vi "MGI Non-Uniform B-Spline.vi"(6 "Weights[]":dbl[](array[numeric])=[0.25, 0.25, 0.25, 0.25, 0.25, 0.25, 0.25, 0.25, 0.25], 7 "Degree":i32=5, 8 "u":dbl=41.7451, 9 "Knot Multiplicities[]":i32[](array[numeric])=[6, 3, 6], 10 "Knots[]":dbl[](array[numeric])=[0.0, 5.69376337762, 41.7451953785], 11 "Control Points[][]":dbl[][](array[numeric])=[[381.5453186035156, -17.001089096069336, 123.35271453857422], [381.5005798339844, -17.00055503845215, 123.34944152832031], [381.4560241699219, -17.000045776367188, 123.34617614746094], [381.1888427734375, -16.99648094177246, 123.32664489746094], [380.8610534667969, -16.992168426513672, 123.30262756347656], [380.5331115722656, -16.987791061401367, 123.27851104736328], [380.2501525878906, -16.984203338623047, 123.2575912475586], [379.96710205078125, -16.980527877807617, 123.23660278320312], [379.68402099609375, -16.976825714111328, 123.21554565429688]]) -> (3 "C(u)":dbl[](array[numeric]))   [LabVIEW 2020]
doc: "Calculate a Non-uniform rational B-Spline curve value. Input is formatted for compatibility with a STEP file (ISO-10303).\n\nAuthored by Thomas E. Henage\nsupport@mooregoodideas.com\nwww.mooregoodideas.com\n\nCopyright (c) 2010, Moore Good Ideas, Inc.\n\nAll rights reserved.\n\nRedistribution and use in source and binary forms, with or without modification, are permitted provided that the following conditions are met:\n\n * Redistributions of source code must retain the above copyright notice, this list of conditions and the following disclaimer.\n * Redistributions in binary form must reproduce the above copyright notice, this list of conditions and the following disclaimer in the documentation and/or other materials provided with the distribution.\n * Neither the name of Moore Good Ideas, Inc. nor the names of its contributors may be used to endorse or promote products derived from this software without specific prior written permission.\n\nTHIS SOFTWARE IS PROVIDED BY THE COPYRIGHT HOLDERS AND CONTRIBUTORS \"AS IS\" AND ANY EXPRESS OR IMPLIED WARRANTIES, INCLUDING, BUT NOT LIMITED TO, THE IMPLIED WARRANTIES OF MERCHANTABILITY AND FITNESS FOR A PARTICULAR PURPOSE ARE DISCLAIMED. IN NO EVENT SHALL THE COPYRIGHT OWNER OR CONTRIBUTORS BE LIABLE FOR ANY DIRECT, INDIRECT, INCIDENTAL, SPECIAL, EXEMPLARY, OR CONSEQUENTIAL DAMAGES (INCLUDING, BUT NOT LIMITED TO, PROCUREMENT OF SUBSTITUTE GOODS OR SERVICES; LOSS OF USE, DATA, OR PROFITS; OR BUSINESS INTERRUPTION) HOWEVER CAUSED AND ON ANY THEORY OF LIABILITY, WHETHER IN CONTRACT, STRICT LIABILITY, OR TORT (INCLUDING NEGLIGENCE OR OTHERWISE) ARISING IN ANY WAY OUT OF THE USE OF THIS SOFTWARE, EVEN IF ADVISED OF THE POSSIBILITY OF SUCH DAMAGE."
panel:
  out "N(i,n,u)":dbl[][](array[numeric])
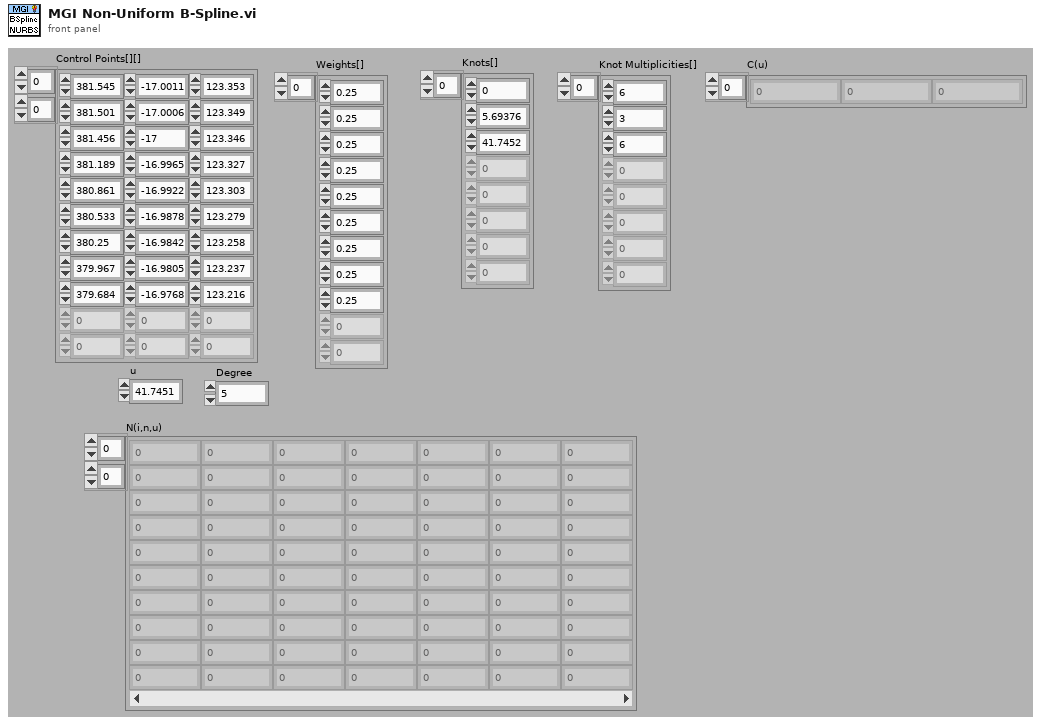
[diagram p1: front panel]
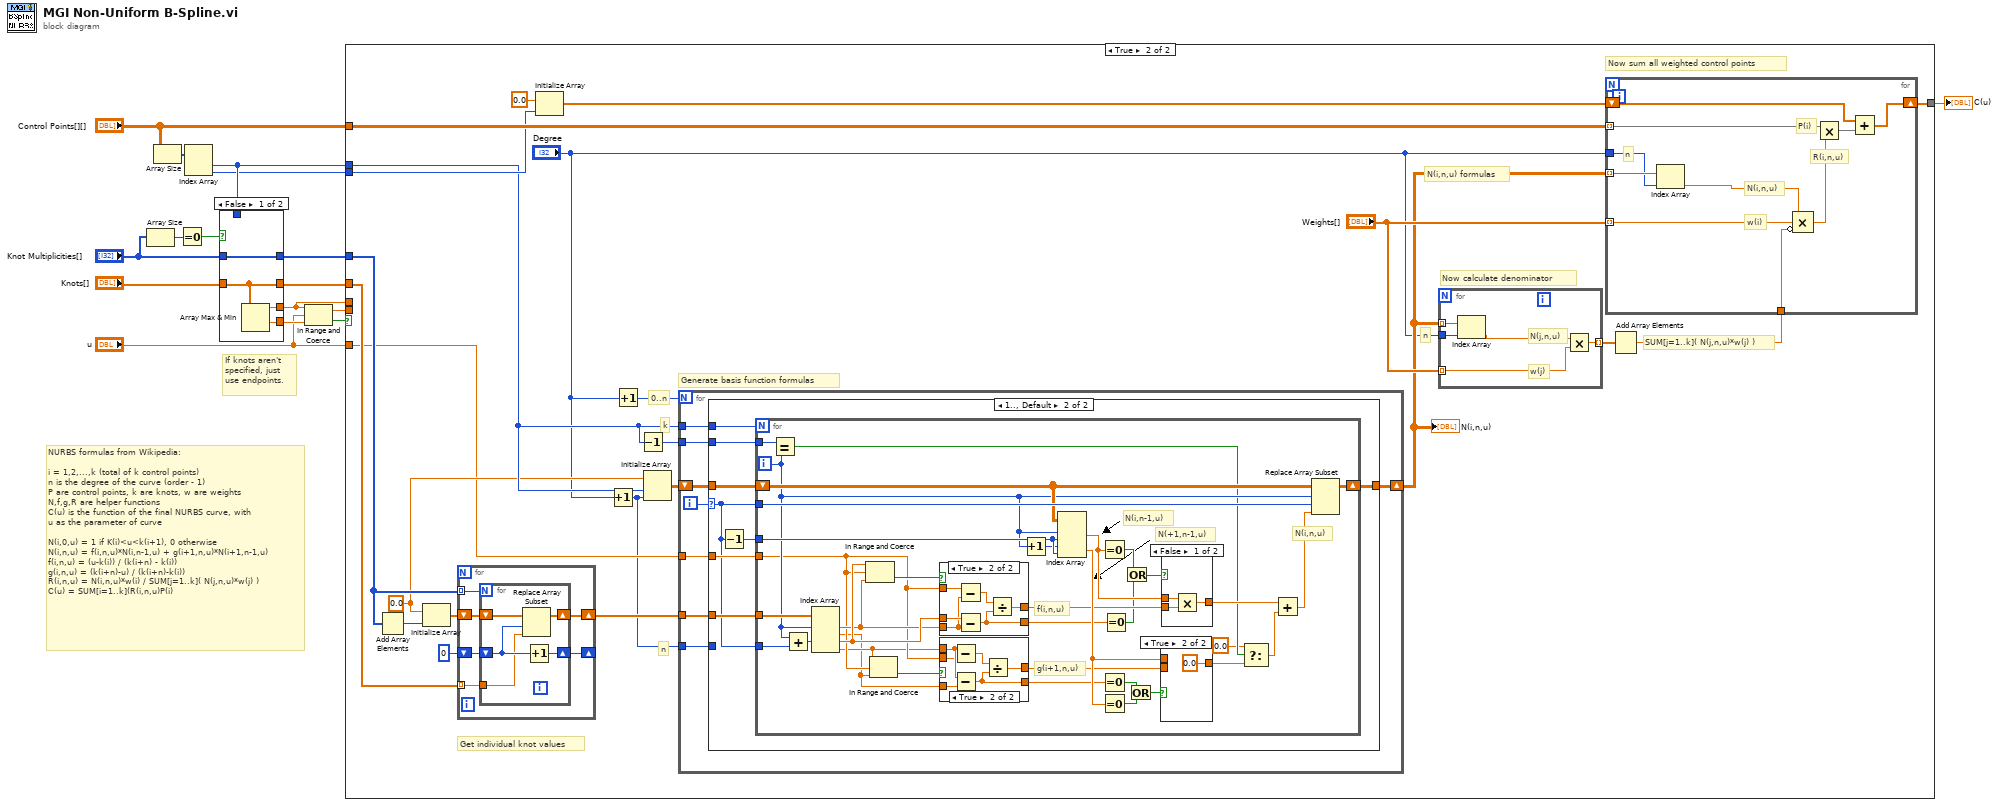
[diagram p0: block diagram]
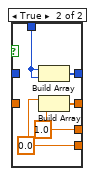
[diagram p2: hidden frame]
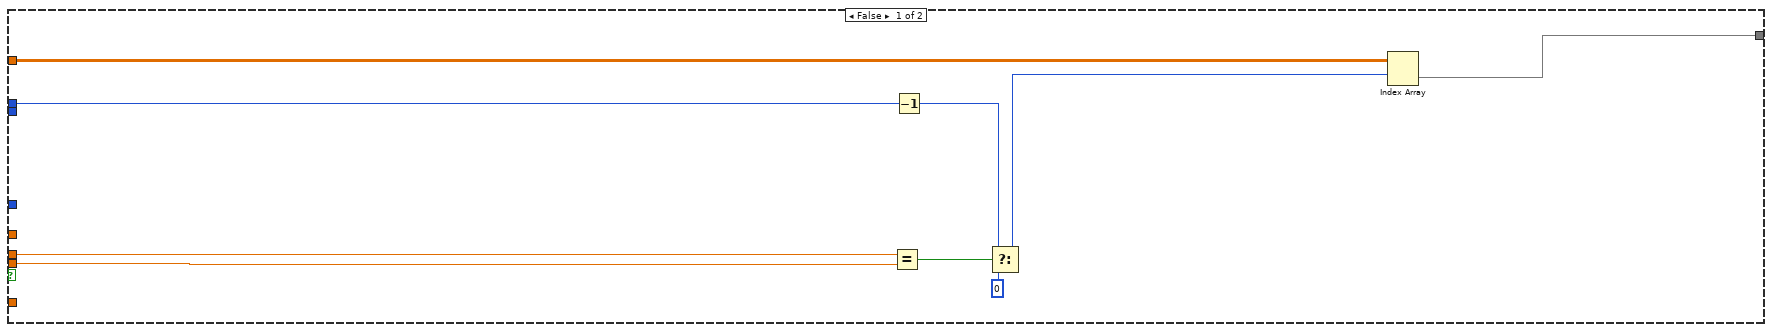
[diagram p3: hidden frame]
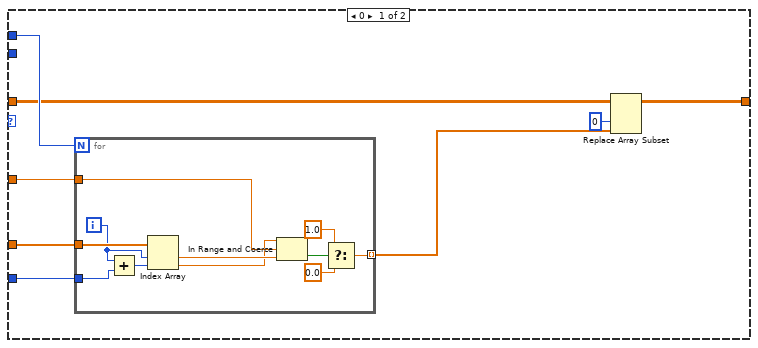
[diagram p4: hidden frame]
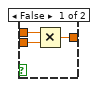
[diagram p7: hidden frame]
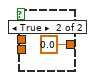
[diagram p8: hidden frame]
diagram:
  # "NURBS formulas from Wikipedia:\n\ni = 1,2,...,k (total of k control points)\nn is the degree of the curve (order - 1)\nP are control points, k are knots, w are weights\nN,f,g,R are helper functions\nC(u) is the function of the final NURBS curve, with\nu as the parameter of curve\n\nN(i,0,u) = 1 if K(i)<u<k(i+1), 0 otherwise\nN(i,n,u) = f(i,n,u)*N(i,n-1,u) + g(i+1,n,u)*N(i+1,n-1,u)\nf(i,n,u) = (u-k(i)) / (k(i+n) - k(i))\ng(i,n,u) = (k(i+n)-u) / (k(i+n)-k(i))\nR(i,n,u) = N(i,n,u)*w(i) / SUM[j=1..k]( N(j,n,u)*w(j) )\nC(u) = SUM[i=1..k](R(i,n,u)P(i)"
  # "If knots aren't\nspecified, just\nuse endpoints."
  n1 = Array Size(array="Knot Multiplicities[]") -> (size(s)=w4:i32)
  n2 = Array Size(array="Control Points[][]") -> (size(s)=w10:i32[])
  n3 = Equal To 0?(x=w4) -> (x = 0?=w3:bool)
  n4 = Index Array(array=w10) -> (element #1=w6:i32, element #2=w2:i32)  [unwired: 2 in]
  n5 = case shown="False" w3 {
    tunnel: "Knots[]" -> [w17 _]
    tunnel: [w20 w24] -> w16
    tunnel: [w19 w25] -> w12
    tunnel: "Knot Multiplicities[]" -> [w18 _]
    tunnel: [w18 w21] -> w8
    tunnel: [w17 w23] -> w7
    tunnel: w6 -> [_ w22]
    frame False {
      n6 = Array Max & Min(array=w17) -> (max value=w19:dbl, min value=w20:dbl)  [unwired: 2 out]
    }
    frame True {
      w24 = 0.0
      w25 = 1.0
      n7 = Build Array(w22, w22) -> (w21:i32[])
      n8 = Build Array(w24, w25) -> (w23:dbl[])
    }
  }
  n9 = In Range and Coerce(upper limit=w12, x="u", lower limit=w16) -> (coerced(x)=w13:dbl, In Range?=w14:bool)
  n10 = case shown="True" w14 {
    tunnel: w7 -> [_ w48]
    tunnel: "u" -> [_ w37]
    tunnel: w13 -> [w34 _]
    tunnel: w12 -> [w33 _]
    tunnel: "Control Points[][]" -> [w32 w57]
    tunnel: [w31 w53] -> w11
    tunnel: w6 -> [w30 w47]
    tunnel: w8 -> [_ w44]
    tunnel: w2 -> [_ w56]
    frame False {
      n11 = Equal?(x=w33, y=w34) -> (x = y?=w29:bool)
      n12 = Decrement(x=w30) -> (x-1=w28:i32)
      n13 = Select(t=w28, s=w29, f=0) -> (s? t:f=w26:i32)
      n14 = Index Array(array=w32, index (row)=w26) -> (element=w31:dbl[])  [unwired: 1 in]
    }
    frame True {
      w38 = 0.0
      # "Get individual knot values"
      # "n"
      # "0..n"
      # "k"
      # "Now sum all weighted control points"
      # "Now calculate denominator"
      # "Generate basis function formulas"
      # "n"
      # "SUM[j=1..k]( N(j,n,u)*w(j) )"
      # "N(i,n,u) formulas"
      n15 = Add Array Elements(numeric array=w44) -> (sum=w42:i32)
      n16 = Initialize Array(w38, w42) -> (w43:dbl[])
      n17 = for {
        tunnel: w48 -> [w63] mode=indexing
        tunnel: w44 -> [w62] mode=indexing
        shift-right: [w60] -> w40
        shift-left: w43 -> [w61]
        shift-right: [w58] -> _
        shift-left: 0 -> [w59]
        n18 = for {
          N: w62 -> [_]
          tunnel: w63 -> [w64]
          shift-right: [w67] -> w60
          shift-left: w61 -> [w68]
          shift-right: [w65] -> w58
          shift-left: w59 -> [w66]
          n19 = Replace Array Subset(array=w68, new element=w64, index=w66) -> (w67:dbl[])
          n20 = Increment(x=w66) -> (x+1=w65:i32)
        }
      }
      n21 = Initialize Array(0.0 ("element"), w56) -> (w54:dbl[])
      n22 = Increment(x="Degree") -> (x+1=w35:i32)
      n23 = Increment(x="Degree") -> (x+1=w45:i32)
      n24 = Decrement(x=w47) -> (x-1=w46:i32)
      n25 = Initialize Array(w38, w47, w35) -> (w49:dbl[][])
      n26 = for {
        N: w45 -> [_]
        shift-right: [w72] -> w39
        shift-left: w49 -> [w75]
        tunnel: w40 -> [w74]
        tunnel: w47 -> [w73]
        tunnel: w46 -> [w71]
        tunnel: w37 -> [w70]
        tunnel: w35 -> [w69]
        i -> [w76]
        n27 = case shown="1.., Default" w76 {
          selector: w76 -> [_ w96]
          tunnel: w75 -> [w81 w103]
          tunnel: w74 -> [w83 w99]
          tunnel: w73 -> [w84 w102]
          tunnel: [w80 w101] -> w72
          tunnel: w71 -> [_ w100]
          tunnel: w70 -> [w82 w97]
          tunnel: w69 -> [w77 _]
          frame 0 {
            n28 = for {
              N: w84 -> [_]
              tunnel: w83 -> [w95]
              tunnel: w77 -> [w94]
              tunnel: w82 -> [w93]
              tunnel: [w87] -> w79 mode=indexing
              i -> [w85]
              n29 = Add(x=w85, y=w94) -> (x+y=w86:i32)
              n30 = Index Array(array=w95, index #1=w85, index #2=w86) -> (element #1=w92:dbl, element #2=w91:dbl)
              n31 = In Range and Coerce(upper limit=w91, x=w93, lower limit=w92) -> (In Range?=w90:bool)  [unwired: 1 out]
              n32 = Select(t=1.0, s=w90, f=0.0) -> (s? t:f=w87:dbl)
            }
            n33 = Replace Array Subset(array=w81, new element=w79, index (col)=0 ("disabled index (col)")) -> (w80:dbl[][])  [unwired: 1 in]
          }
          frame 1.., Default {
            n34 = Decrement(x=w96) -> (x-1=w98:i32)
            n35 = for {
              N: w102 -> [_]
              shift-right: [w135] -> w101
              shift-left: w103 -> [w133]
              tunnel: w100 -> [w138]
              tunnel: w99 -> [w137]
              tunnel: w96 -> [w134]
              tunnel: w98 -> [w132]
              tunnel: w96 -> [w129]
              tunnel: w97 -> [w107]
              i -> [w131]
              # "g(i+1,n,u)"
              # "f(i,n,u)"
              # "N(+1,n-1,u)"
              # "N(i,n,u)"
              # "N(i,n-1,u)"
              n36 = Equal?(x=w138, y=w131) -> (x = y?=w125:bool)
              n37 = Add(x=w131, y=w129) -> (x+y=w136:i32)
              n38 = Index Array(array=w137, index #1=w131, index #3=w136) -> (element #1=w109:dbl, element #2=w105:dbl, element #3=w110:dbl, element #4=w106:dbl)  [unwired: 2 in]
              n39 = In Range and Coerce(upper limit=w110, x=w107, lower limit=w109) -> (In Range?=w108:bool)  [unwired: 1 out]
              n40 = In Range and Coerce(upper limit=w106, x=w107, lower limit=w105) -> (In Range?=w104:bool)  [unwired: 1 out]
              n41 = case shown="True" w108 {
                tunnel: [_ w149] -> w118
                tunnel: [_ w148] -> w112
                tunnel: w107 -> [_ w147]
                tunnel: w110 -> [_ w146]
                tunnel: w109 -> [_ w145]
                frame False {
                }
                frame True {
                  n42 = Subtract(x=w147, y=w145) -> (x-y=w150:dbl)
                  n43 = Subtract(x=w146, y=w145) -> (x-y=w148:dbl)
                  n44 = Divide(x=w150, y=w148) -> (x/y=w149:dbl)
                }
              }
              n45 = case shown="True" w104 {
                tunnel: w106 -> [_ w144]
                tunnel: w105 -> [_ w143]
                tunnel: [_ w141] -> w115
                tunnel: [_ w140] -> w111
                tunnel: w107 -> [_ w139]
                frame False {
                }
                frame True {
                  n46 = Subtract(x=w144, y=w139) -> (x-y=w142:dbl)
                  n47 = Subtract(x=w144, y=w143) -> (x-y=w140:dbl)
                  n48 = Divide(x=w142, y=w140) -> (x/y=w141:dbl)
                }
              }
              n49 = Increment(x=w131) -> (x+1=w130:i32)
              n50 = Index Array(array=w133, index (row) #1=w131, index (col) #1=w132, index (row) #2=w130, index (col) #2=w132) -> (element #1=w122:dbl, element #2=w119:dbl)
              n51 = Equal To 0?(x=w122) -> (x = 0?=w121:bool)
              n52 = Equal To 0?(x=w111) -> (x = 0?=w113:bool)
              n53 = Equal To 0?(x=w119) -> (x = 0?=w120:bool)
              n54 = Equal To 0?(x=w112) -> (x = 0?=w116:bool)
              n55 = Or(x=w121, y=w116) -> (x .or. y?=w117:bool)
              n56 = Or(x=w113, y=w120) -> (x .or. y?=w114:bool)
              n57 = case shown="True" w114 {
                tunnel: w115 -> [w153 _]
                tunnel: w119 -> [w152 _]
                tunnel: [w151 0.0] -> w126
                frame False {
                  n58 = Multiply(x=w152, y=w153) -> (x*y=w151:dbl)
                }
                frame True {
                }
              }
              n59 = case shown="False" w117 {
                tunnel: w118 -> [w157 _]
                tunnel: w122 -> [w156 _]
                tunnel: [w155 0.0] -> w128
                frame False {
                  n60 = Multiply(x=w156, y=w157) -> (x*y=w155:dbl)
                }
                frame True {
                }
              }
              n61 = Select(t=0.0, s=w125, f=w126) -> (s? t:f=w123:dbl)
              n62 = Add(x=w128, y=w123) -> (x+y=w127:dbl)
              n63 = Replace Array Subset(array=w133, new element=w127, index (row)=w131, index (col)=w134) -> (w135:dbl[][])
            }
          }
        }
      }
      "N(i,n,u)" <- w39
      n64 = for {
        tunnel: w39 -> [w163] mode=indexing
        tunnel: "Weights[]" -> [w160] mode=indexing
        tunnel: "Degree" -> [w162]
        tunnel: [w161] -> w52 mode=indexing
        # "w(j)"
        # "N(j,n,u)"
        n65 = Index Array(array=w163, index=w162) -> (element=w159:dbl)
        n66 = Multiply(x=w159, y=w160) -> (x*y=w161:dbl)
      }
      n67 = Add Array Elements(numeric array=w52) -> (sum=w50:dbl)
      n68 = for {
        tunnel: w57 -> [w170] mode=indexing
        shift-right: [w171] -> w53
        shift-left: w54 -> [w172]
        tunnel: "Weights[]" -> [w167] mode=indexing
        tunnel: "Degree" -> [w166]
        tunnel: w39 -> [w168] mode=indexing
        tunnel: w50 -> [w165]
        # "n"
        # "w(i)"
        # "N(i,n,u)"
        # "R(i,n,u)"
        # "P(i)"
        n69 = Index Array(array=w168, index=w166) -> (element=w164:dbl)
        n70 = Compound Arithmetic op=MULTIPLY(w164, w167, invert w165) -> (w169:dbl)
        n71 = Multiply(x=w170, y=w169) -> (x*y=w173:dbl[])
        n72 = Add(x=w172, y=w173) -> (x+y=w171:dbl[])
      }
    }
  }
  "C(u)" <- w11
